vi "Constants.vi"() -> ()   [LabVIEW 2018]
panel:
  in  "Turn Travel\nUnits Per Rotation":dbl=3600.0
  in  "Rotations\nTo Travel":dbl=6.0
  in  "Position High Gains":T1={"kP"=0.56, "kI "=0.0, "kD"=0.001, "kF"=0.15, "I Zone"=400.0, "Peak Out"=1.0}
  in  "Position Low Gains":T1={"kP"=0.23, "kI "=0.0, "kD"=0.005, "kF"=0.12, "I Zone"=300.0, "Peak Out"=1.0}
  in  "Turn High Gains":T1={"kP"=3.4, "kI "=0.0, "kD"=1.0, "kF"=0.0, "I Zone"=200.0, "Peak Out"=1.0}
  in  "Turn Low Gains":T1={"kP"=3.5, "kI "=0.0, "kD"=3.0, "kF"=0.0, "I Zone"=100.0, "Peak Out"=1.0}
  in  "Neutral\nDeadband":dbl=0.001
  in  "Timeout Ms":i32=10
  in  "Pigeon Units\nPer Rotatoin":i32=8192
  in  "Encoder Units\nPer Rotation":i32=51711
  in  "Heading Sensor\nChoice":i32
  in  "Sensor Units\nPer Rotation":i32=4096
  in  "Turn Low Gains Slot":i32=3
  in  "Position Low Gains Slot":i32=2
  in  "Turn High Gains Slot":i32=1
  in  "Position High Gains Slot":i32
  in  "PID Turn":i32=1
  in  "PID Primary":i32
  in  "REMOTE 1":i32=1
  in  "REMOTE 0":i32
  # "How many\nsensor units\nper rotation:\nCTRE Mag\nEncoder"
  # "How to measure\nrobot heading:\n0 - Diff b/w left & right\n1 - Pigeon IMU"
  # "Empirically\nmeasure the\ndifference\nbetween \nencoders per\n360 degrees"
  # "Scales units to\n3600 per rotation.\nThis is nice, as it\nmeans one unit is\n0.1 degrees."
  # "Property of pigeon\nshould not be\nchanged"
  # "Constants"
  # "You shouldn't need\nto change these"
  # "0 - Skip confirmation\nNonZero - Wait and log\nto DS if something fails"
  # "Motor's\nNeutral deadband"
  # "0.1411423841 = 1023/7248"
  # "1023 = Max Output\n7248 = Measured Max Output"
  # "max speed in low gear: 100 in/s"
  # "max speed in low gear: 8104 su/idk"
  # "7319 speed on ground high gear: 0.13977"
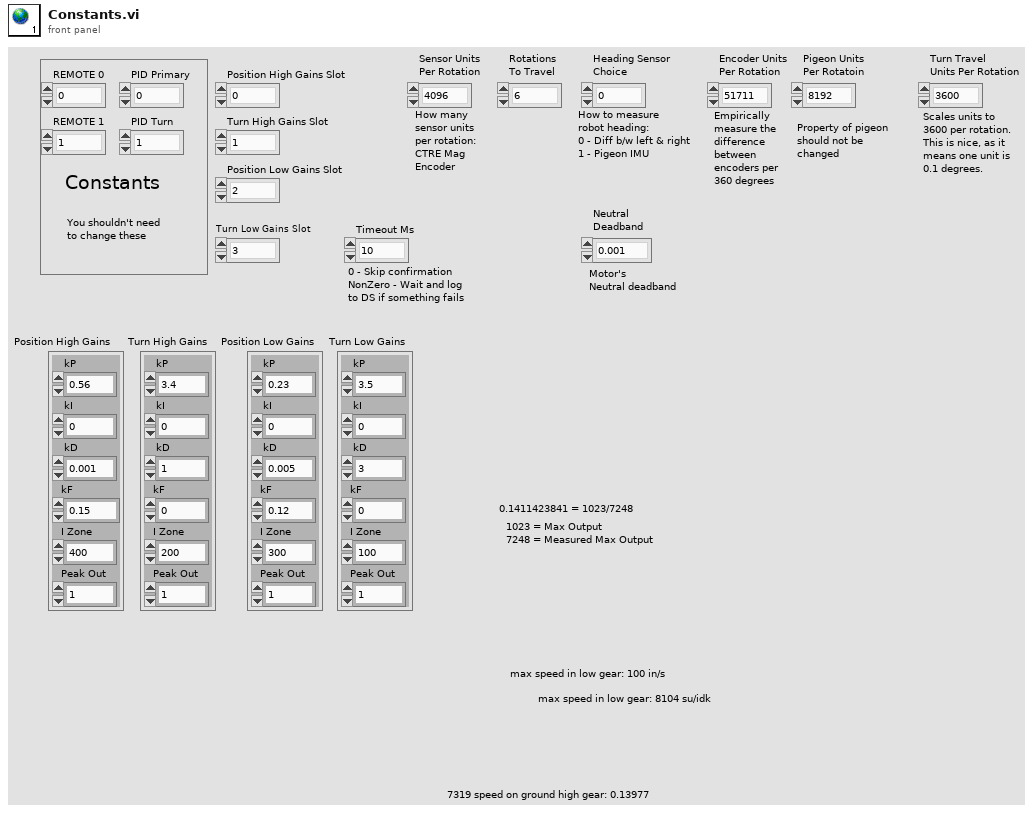
[diagram p1: front panel]
types:
  T1 = cluster{"kP":dbl, "kI ":dbl, "kD":dbl, "kF":dbl, "I Zone":dbl, "Peak Out":dbl}
diagram:
